vi "DATADYNTESTmonoligne.vi"(8 "errin":errorcluster, 9 "SN":string="0B5MEVA000CA1JC1M0000041", 10 "Limites":T1, 11 "visain":refnum<visa-resource-name>) -> (0 "errout":errorcluster, 2 "chaîne concaténée":string, 3 "visaout":refnum<visa-resource-name>)   [LabVIEW 2020]
doc: "Test et trace en BDD l'OCV et les V/TCell"
uses:
  <vilib>/addons/database/Connection.llb/DB Tools Open Connec (String).vi
  <vilib>/addons/database/Connection.llb/Conn Execute.vi
  <vilib>/addons/database/Recordset.llb/Rec Destroy - Connection.vi
  <vilib>/addons/database/NI_Database_API.lvlib
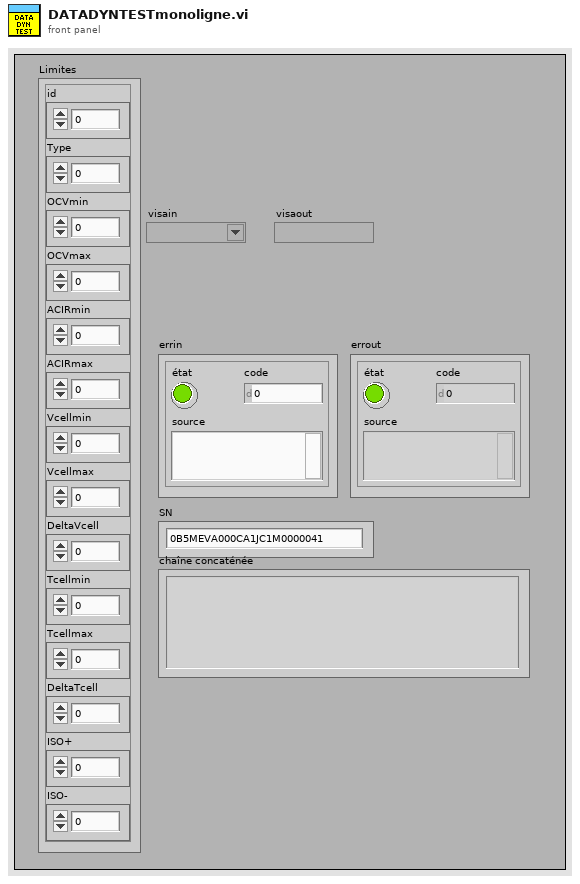
[diagram p1: front panel]
types:
  T1 = cluster{"id":dbl, "Type":dbl, "OCVmin":dbl, "OCVmax":dbl, "ACIRmin":dbl, "ACIRmax":dbl, "Vcellmin":dbl, "Vcellmax":dbl, "DeltaVcell":dbl, "Tcellmin":dbl, "Tcellmax":dbl, "DeltaTcell":dbl, "ISO+":dbl, "ISO-":dbl}
  T2 = cluster{"Cell1 V":sgl, "Cell2 V":sgl, "Cell3 V":sgl, "Cell4 V":sgl, "Cell1 °C":sgl, "Cell2 °C":sgl, "Cell5 V":sgl, "Cell6 V":sgl}
  T3 = typedef "NI_Database_API.lvlib/Conn ObjectReference.ctl" = refnum<k1>
  T4 = typedef "NI_Database_API.lvlib/Rec ObjectReference.ctl" = refnum<k1>
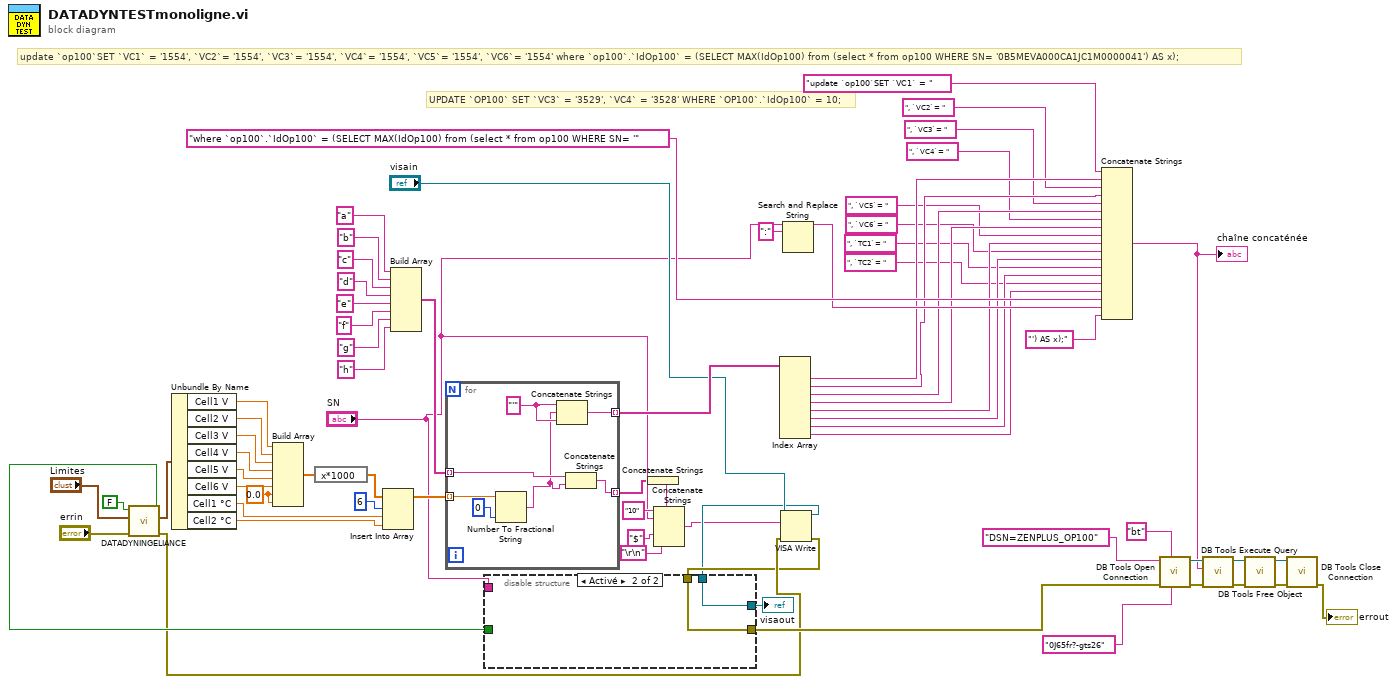
[diagram p0: block diagram]
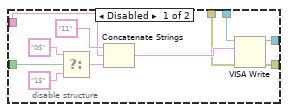
[diagram p2: hidden frame]
diagram:
  w47 = sgl 0.0 ("élément")
  # "update `op100`SET `VC1` = '1554', `VC2`= '1554', `VC3`= '1554', `VC4`= '1554', `VC5`= '1554', `VC6`= '1554' where `op100`.`IdOp100` = (SELECT MAX(IdOp100) from (select * from op100 WHERE SN= '0B5MEVA000CA1JC1M0000041') AS x);"
  # "UPDATE `OP100` SET `VC3` = '3529', `VC4` = '3528' WHERE `OP100`.`IdOp100` = 10;"
  n1 = call "DATADYNINGELIANCE.vi"("errin"="errin", "Limites"="Limites", "3P4S"=FALSE) -> ("errout"=w11:errorcluster, "Out"=w50:T2, "test OK?"=w46:bool)  [unwired: 4 in, 2 out]
  n2 = Unbundle By Name(w50) -> ("Cell1 V"=w60:sgl, "Cell2 V"=w61:sgl, "Cell3 V"=w62:sgl, "Cell4 V"=w63:sgl, "Cell5 V"=w64:sgl, "Cell6 V"=w65:sgl, "Cell1 °C"=w69:sgl, "Cell2 °C"=w70:sgl)
  n3 = Build Array(w60, w61, w62, w63, w64, w65, w47, w47) -> (w66:sgl[])
  n4 = expression code="x*1000"(w66) -> (w67:sgl[])
  n5 = Insert Into Array(array=w67, index=6 ("indice"), new element #1=w69, new element #2=w70) -> (w71:sgl[])
  n6 = Build Array("a", "b", "c", "d", "e", "f", "g", "h") -> (w59:string[])
  n7 = for {
    tunnel: w59 -> [w79] mode=indexing
    tunnel: w71 -> [w78] mode=indexing
    tunnel: [w75] -> w30 mode=indexing
    tunnel: [w73] -> w3 mode=indexing
    w76 = "'" ("chaîne")
    n8 = Number To Fractional String ("Nombre en chaîne fractionnaire")(number=w78, precision (6)=i16 0 ("précision (6)")) -> (F-format string=w74:string)  [unwired: 2 in]
    n9 = Concatenate Strings(w76, w74, w76) -> (w75:string)
    n10 = Concatenate Strings(w79, w74) -> (w73:string)
  }
  n11 = Concatenate Strings(w3) -> (w2:string)
  n12 = Concatenate Strings("10" ("chaîne"), "SN", w2, "$" ("chaîne"), "\r\n") -> (w1:string)
  n13 = Index Array(array=w30) -> (element #1=w29:string, element #2=w27:string, element #3=w25:string, element #4=w23:string, element #5=w21:string, element #6=w19:string, element #7=w15:string, element #8=w12:string)  [unwired: 8 in]
  n14 = VISA Write(VISA resource name="visain", write buffer=w1, error in (no error)=w11) -> (VISA resource name out=w8:refnum<visa-resource-name>, error out=w9:errorcluster)  [unwired: 1 out]
  n15 = disable-structure shown="Activé" {
    disable-tunnel: w46 -> [w86 _]
    disable-tunnel: "SN" -> [w85 _]
    disable-tunnel: w8 -> [w83 w92]
    disable-tunnel: [w82 w92] -> w45
    disable-tunnel: [w81 w91] -> w17
    disable-tunnel: w9 -> [w80 w91]
    frame Disabled {
      n16 = Select(t="0$" ("chaîne"), s=w86, f="1$" ("chaîne")) -> (s? t:f=w87:string)
      n17 = Concatenate Strings("11" ("chaîne"), w85, w87) -> (w84:string)
      n18 = VISA Write(VISA resource name=w83, write buffer=w84, error in (no error)=w80) -> (VISA resource name out=w82:refnum<visa-resource-name>, error out=w81:errorcluster)  [unwired: 1 out]
    }
    frame Enabled {
    }
  }
  "visaout" <- w45
  n19 = Search and Replace String ("Rechercher et remplacer une chaîne")(input string="SN", search string=":" ("chaîne recherchée")) -> (result string=w32:string)  [unwired: 6 in, 3 out]
  n20 = Concatenate Strings("update `op100`SET `VC1` = " ("chaîne"), w29, ", `VC2`= " ("chaîne"), w27, ", `VC3`= " ("chaîne"), w25, ", `VC4`= " ("chaîne"), w23, ", `VC5`= " ("chaîne"), w21, ", `VC6`= " ("chaîne"), w19, ", `TC1`= " ("chaîne"), w15, ", `TC2`= " ("chaîne"), w12, "where `op100`.`IdOp100` = (SELECT MAX(IdOp100) from (select * from op100 WHERE SN= '" ("chaîne"), w32, "') AS x);" ("chaîne")) -> (w39:string)
  "chaîne concaténée" <- w39
  n21 = call-poly <vilib>:"DB Tools Open Connection.vi"("password"="0J65fr?-gts26", "userID"="bt", "error in (no error)"=w17, "connection information"="DSN=ZENPLUS_OP100") -> ("error out"=w44:errorcluster, "connection reference"=w42:T3)  [unwired: 4 in]
  n22 = call-poly <vilib>:"DB Tools Execute Query.vi"("error in (no error)"=w44, "SQL query"=w39, "connection reference"=w42) -> ("error out"=w35:errorcluster, "recordset reference"=w34:T4)  [unwired: 5 in]
  n23 = call-poly <vilib>:"DB Tools Free Object.vi"("error in (no error)"=w35, "recordset reference"=w34) -> ("error out"=w43:errorcluster, "connection reference"=w41:T3)  [unwired: 8 in]
  n24 = call <vilib>:"DB Tools Close Connection.vi"("error in (no error)"=w43, "connection reference"=w41) -> ("error out"=→"errout":errorcluster)  [unwired: 5 in]
